vi "Puff_using_Arduino_oneshot.vi"(0 "Puff_duration:Sec":dbl=1.0 format="%.2g") -> ()   [LabVIEW 2017]
uses:
  Controls/Post_Process.ctl
  Controls/Setup.ctl
  Globals/Meas_global.vi
panel:
  out "Puff Time used":dbl=1.0 format="%.2g"
  out "Case Currently On":string="Loop"
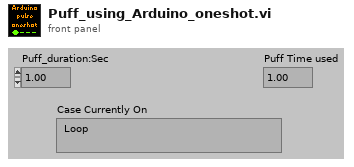
[diagram p1: front panel]
types:
  T1 = typedef "Setup.ctl" = enum16{"Run Program", "Show Setup", "Save Current Setup", "Setup Front Panel"}
  T2 = typedef "Post_Process.ctl" = enum16{"Take New Data", "Post Process Raw Data File"}
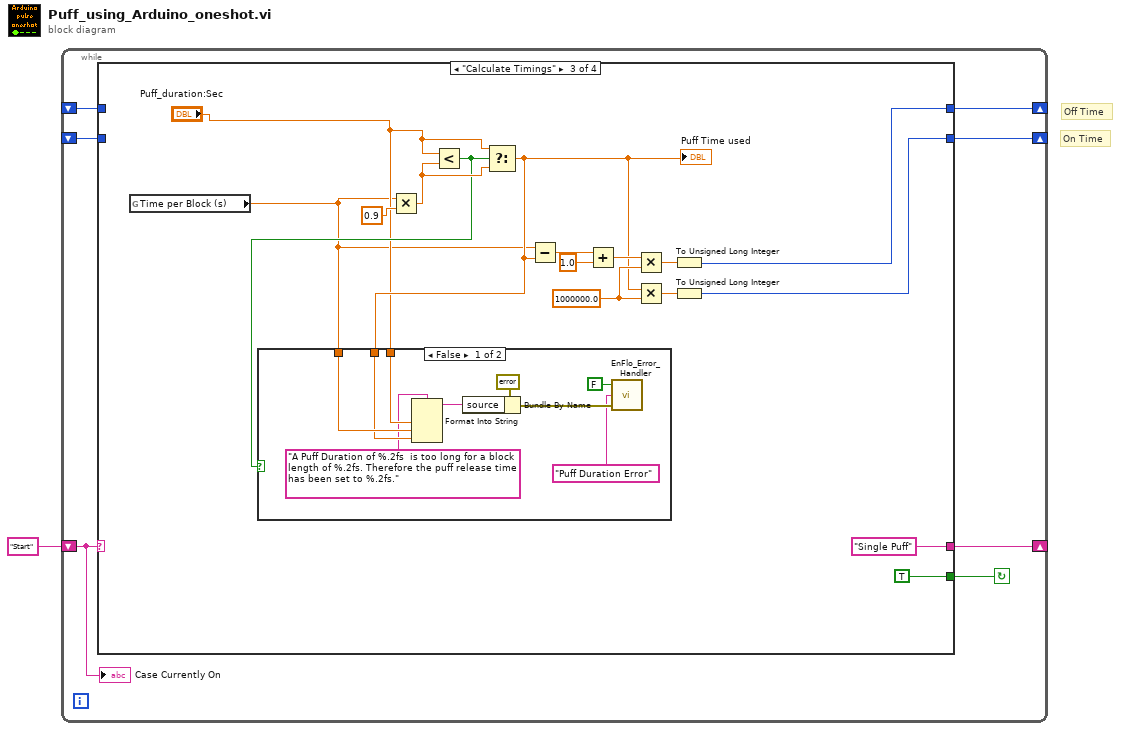
[diagram p0: block diagram]
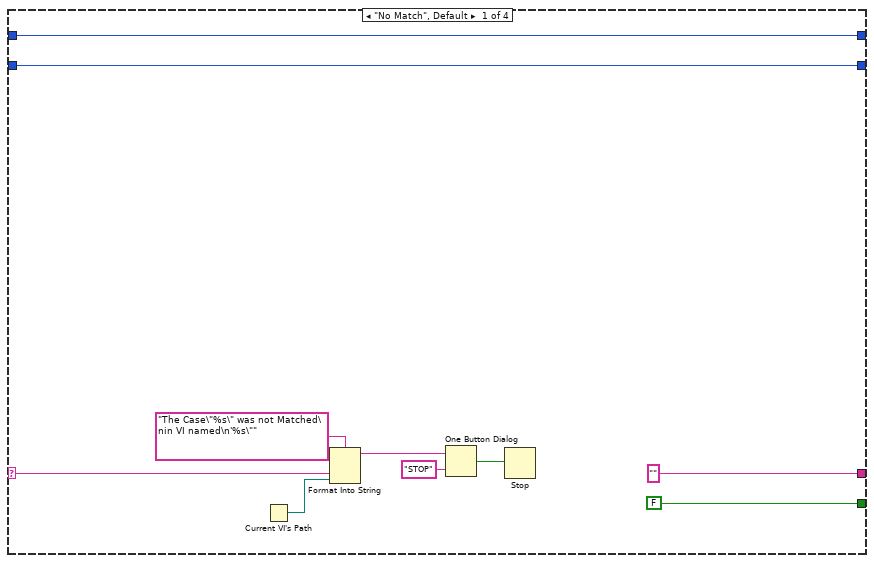
[diagram p2: hidden frame]
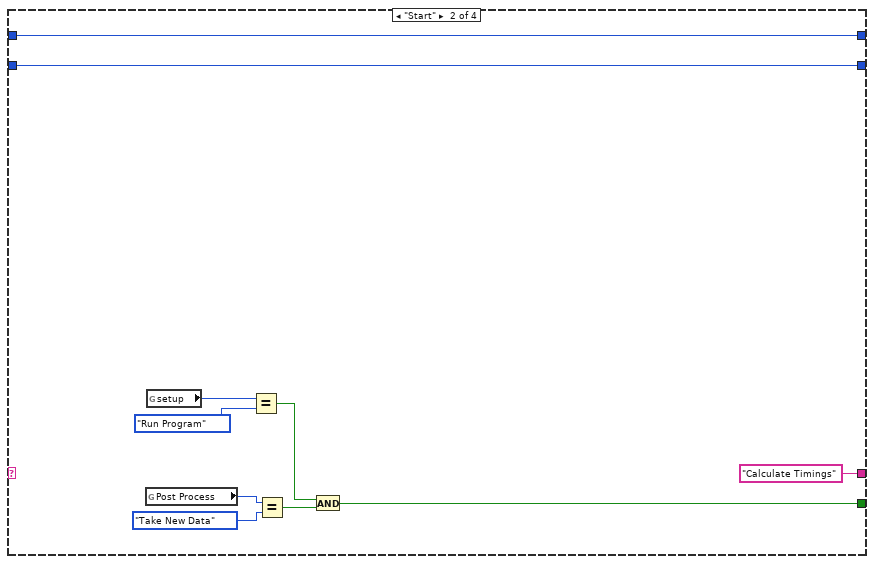
[diagram p3: hidden frame]
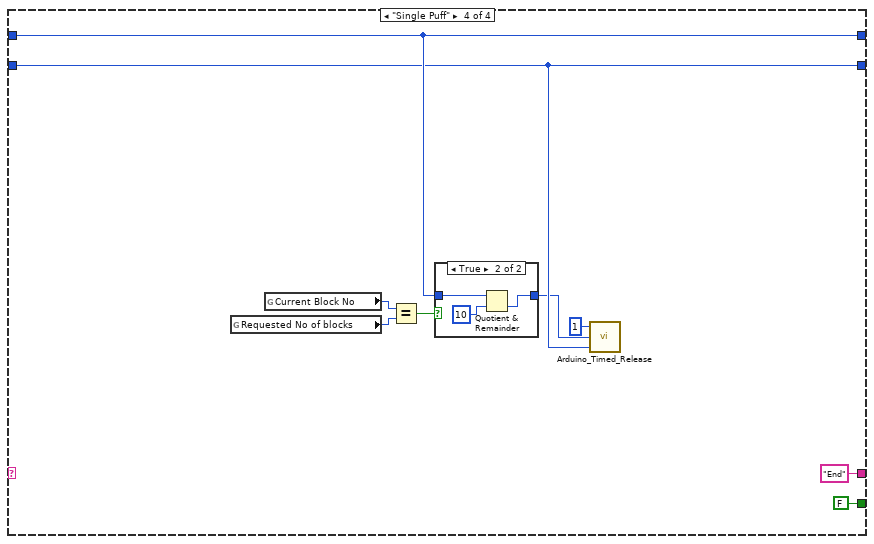
[diagram p5: hidden frame]
diagram:
  # "On Time"
  # "Off Time"
  n1 = while {
    shift-left: "Start" -> [w6]
    shift-right: [w7] -> _
    shift-right: [w5] -> _
    shift-left: _ -> [w4]
    shift-right: [w3] -> _
    shift-left: _ -> [w2]
    stop <- w8 continue-if-true
    n2 = case shown="\"Calculate Timings\"" w6 {
      selector: w6 -> [w9 _ _ _]
      tunnel: [FALSE w21 TRUE ("Command Found") FALSE ("Command Found")] -> w8
      tunnel: ["" "Calculate Timings" "Single Puff" "End"] -> w7
      tunnel: [w11 w20 w32 w62] -> w5
      tunnel: w4 -> [w11 w20 _ w62]
      tunnel: [w10 w19 w31 w61] -> w3
      tunnel: w2 -> [w10 w19 _ w61]
      frame "No Match", Default {
        n3 = Current VI's Path() -> (path=w13:path)
        n4 = Format Into String(format string="The Case\"%s\" was not Matched\nin VI named\n'%s\"" ("Format String"), w9, w13) -> (resulting string=w16:string)  [unwired: 2 in, 1 out]
        n5 = One Button Dialog(message=w16, button name ("OK")="STOP") -> (true=w14:bool)
        n6 = Stop(stop? (T)=w14) -> ()
      }
      frame "Start" {
        n7 = global read "Meas_global.vi" "Post Process"() -> (w23:T2)
        n8 = global read "Meas_global.vi" "setup"() -> (w22:T1)
        n9 = Equal?(x=w22, y=Setup."Run Program") -> (x = y?=w27:bool)
        n10 = Equal?(x=w23, y=Post_Process."Take New Data" ("Post Process")) -> (x = y?=w26:bool)
        n11 = And(x=w27, y=w26) -> (x .and. y?=w21:bool)
      }
      frame "Calculate Timings" {
        w38 = 1000000.0 ("y")
        n12 = global read "Meas_global.vi" "Time per Block (s)"() -> (w29:dbl)
        n13 = Multiply(x=w29, y=0.9) -> (x*y=w41:dbl)
        n14 = Less?(x="Puff_duration:Sec", y=w41) -> (x < y?=w34:bool)
        n15 = Select(t="Puff_duration:Sec", s=w34, f=w41) -> (s? t:f=w33:dbl)
        "Puff Time used" <- w33
        n16 = case shown="False" w34 {
          tunnel: "Puff_duration:Sec" -> [w51 _]
          tunnel: w29 -> [w50 _]
          tunnel: w33 -> [w49 _]
          frame False {
            n17 = Format Into String(format string="A Puff Duration of %.2fs  is too long for a block length of %.2fs. Therefore the puff release time has been set to %.2fs.", w51, w50, w49) -> (resulting string=w47:string)  [unwired: 2 in, 1 out]
            n18 = Bundle By Name(cluster=errorcluster {"status"=TRUE, "code"=0, "source"=""} ("error in (no error)"), "source"=w47) -> (w52:errorcluster)
            n19 = call "EnFlo_Error_Handler.vi"("error in (no error)"=w52, "Error Type"="Puff Duration Error", "Dialog Box (T)"=FALSE) -> ()  [unwired: 3 out]
          }
          frame True {
          }
        }
        n20 = Subtract(x=w29, y=w33) -> (x-y=w37:dbl)
        n21 = Add(x=w37, y=1.0) -> (x+y=w35:dbl)
        n22 = Multiply(x=w35, y=w38) -> (x*y=w39:dbl)
        n23 = Multiply(x=w33, y=w38) -> (x*y=w40:dbl)
        n24 = To Unsigned Long Integer(number=w39) -> (unsigned 32bit integer=w32:u32)
        n25 = To Unsigned Long Integer(number=w40) -> (unsigned 32bit integer=w31:u32)
      }
      frame "Single Puff" {
        n26 = global read "Meas_global.vi" "Requested No of blocks"() -> (w56:i32)
        n27 = global read "Meas_global.vi" "Current Block No"() -> (w55:i32)
        n28 = Equal?(x=w55, y=w56) -> (x = y?=w54:bool)
        n29 = case shown="True" w54 {
          tunnel: w62 -> [w63 w66]
          tunnel: [w63 w64] -> w57
          frame False {
          }
          frame True {
            n30 = Quotient & Remainder(x=w66, y=u32 10) -> (floor(x/y)=w64:u32)  [unwired: 1 out]
          }
        }
        n31 = call "Arduino_Timed_Release.vi"("Time to hold source ON (microseconds)"=w61, "Time to hold source OFF (microseconds)"=w57, "Number of cycles"=u16 1) -> ()  [unwired: 2 out]
      }
    }
    "Case Currently On" <- w6
  }
